vi "Get Waveform Data.vi"(8 "error in (no error)":errorcluster, 10 "Waveform to Retrieve":string, 11 "QPA Measurement in":refnum<class "QPA Measurement.lvclass">=refnum) -> (0 "error out":errorcluster, 2 "RF Waveform":T1, 3 "QPA Measurement out":refnum<class "QPA Measurement.lvclass">)   [LabVIEW 2016, in "QPA Measurement.lvlib" / "QPA Measurement.lvclass"]
uses:
  QPA Measurement.lvclass
  Waveform Manager/QPA MSMT Waveform Manager.lvclass
  Waveform Manager/Controls/RF Waveform.ctl
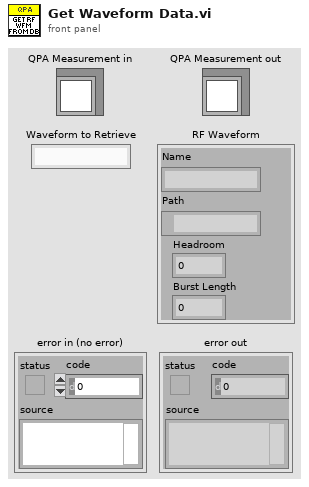
[diagram p1: front panel]
types:
  T1 = typedef "QPA MSMT Waveform Manager.lvclass/RF Waveform.ctl" = cluster{"Name":string, "Path":path, "Headroom":dbl, "Burst Length":dbl}
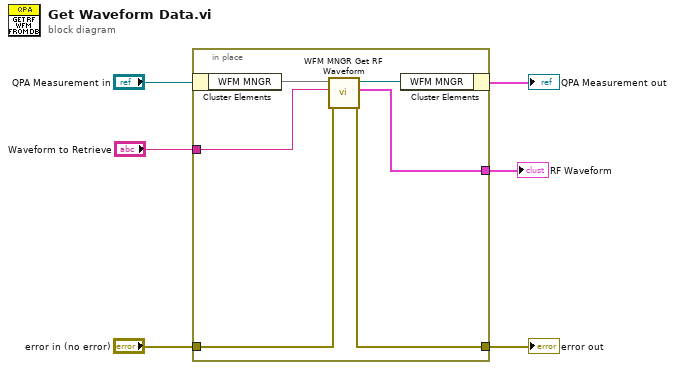
[diagram p0: block diagram]
diagram:
  n1 = in-place {
    in-place-border: "error in (no error)" -> [w10]
    in-place-border: [w9] -> w3
    in-place-border: "Waveform to Retrieve" -> [w8]
    in-place-border: [w7] -> w1
    n2 = in-place-cluster #1("QPA Measurement in") -> ("WFM MNGR"=w12)
    n3 = call "WFM MNGR Get RF Waveform.vi"("error in (no error)"=w10, "Waveform to Retrieve"=w8, "WFM MNGR in"=w12) -> ("error out"=w9:errorcluster, "RF Waveform"=w7:T1, "WFM MNGR out"=w11:refnum<class "QPA MSMT Waveform Manager.lvclass">)  [unwired: 6 in]
    n4 = in-place-cluster #1("WFM MNGR"=w11) -> (→"QPA Measurement out":cluster{})
  }
  "error out" <- w3
  "RF Waveform" <- w1
